vi "Update Control.vi"(8 "error in (no error)":errorcluster, 10 "Ctl Refnum":refnum<vi>, 11 "ControlBindingPanel in":refnum<class "ControlBindingPanel.lvclass">) -> (0 "error out":errorcluster, 3 "ControlBindingPanel out":refnum<class "ControlBindingPanel.lvclass">)   [LabVIEW 2020, in "VolatusGUIEditor.lvlib" / "ControlBindingPanel.lvclass"]
uses:
  ControlBindingPanel.lvclass
  ControlBindingPanel.lvclass/ControlBindingPanel.ctl
  Update Control Data.ctl
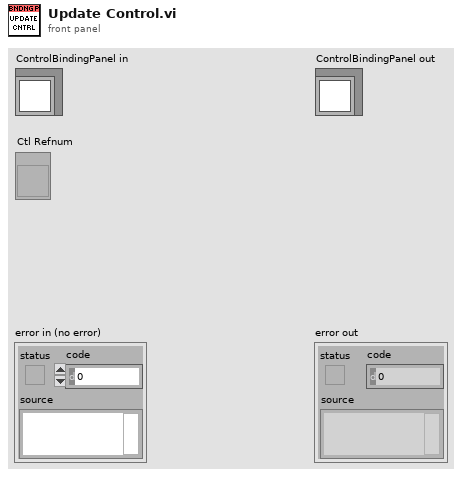
[diagram p1: front panel]
types:
  T1 = typedef "VolatusGUIEditor.lvlib/ControlBindingPanel.lvclass/Update Control Data.ctl" = cluster{"Control":refnum<vi>}
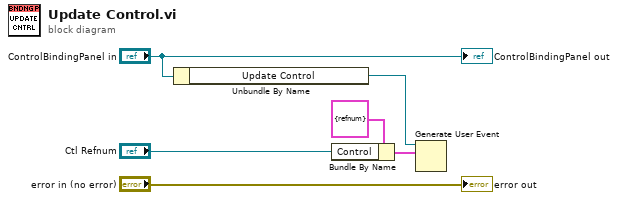
[diagram p0: block diagram]
diagram:
  n1 = Unbundle By Name("ControlBindingPanel in") -> ("Update Control"=w4:refnum<user-event>)
  n2 = Bundle By Name(cluster=T1 {"Control"=refnum} ("event data"), "Control"="Ctl Refnum") -> (w2:T1)
  n3 = Generate User Event(user event=w4, event data cluster=w2) -> ()  [unwired: 2 in, 2 out]
  "error out" <- "error in (no error)"
  "ControlBindingPanel out" <- "ControlBindingPanel in"
